vi "Error Query.vi"(0 "VISA Resource In":refnum<visa-resource-name>, 11 "error in (no error)":errorcluster) -> (4 "VISA Resource Out (dupl)":refnum<visa-resource-name>, 6 "Error Code":i32[](array[numeric]), 8 "Error Message":string, 15 "error out":errorcluster)   [LabVIEW 2025, in "My Current Source.lvlib"]
doc: "Queries the instrument for any errors in the instrument's error queue. It will continue to read errors until all errors have been read from the instrument. Any errors will be returned in the error out indicator."
uses:
  My Current Source.lvlib
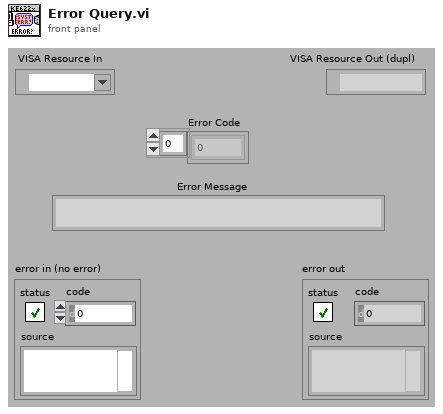
[diagram p1: front panel]
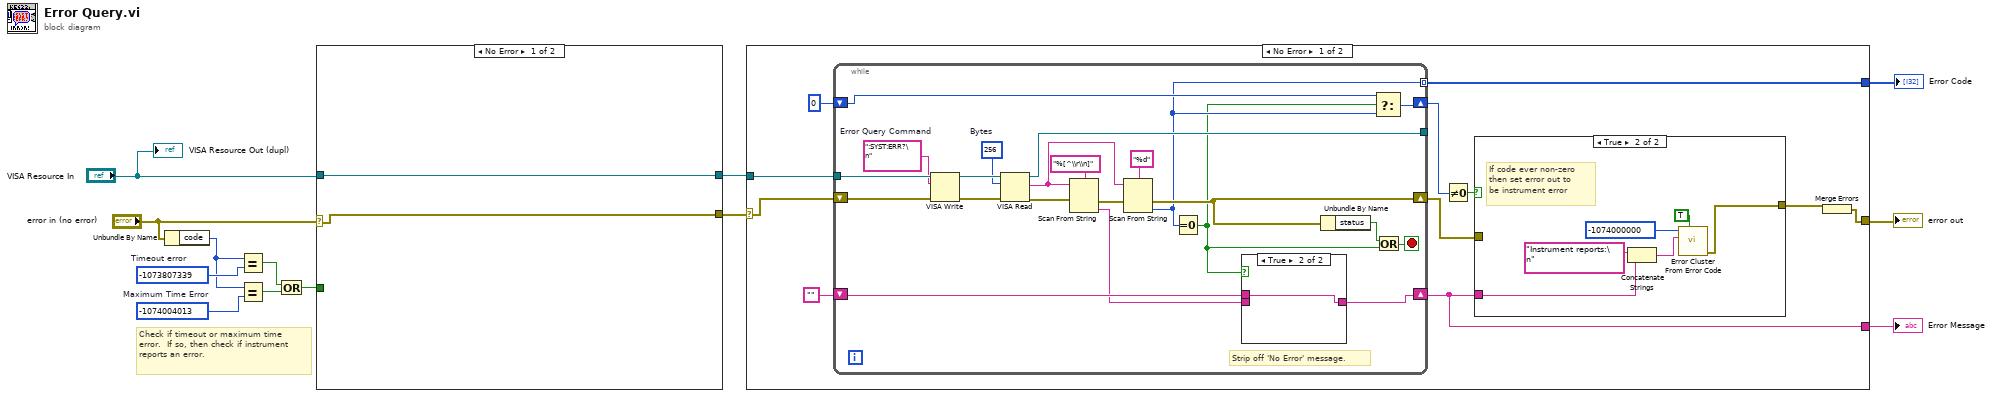
[diagram p0: block diagram]
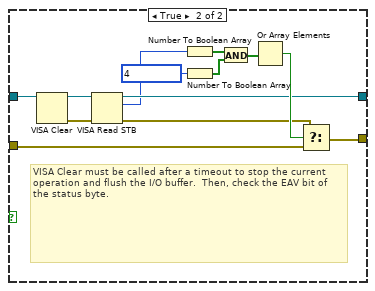
[diagram p3: hidden frame]
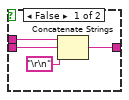
[diagram p5: hidden frame]
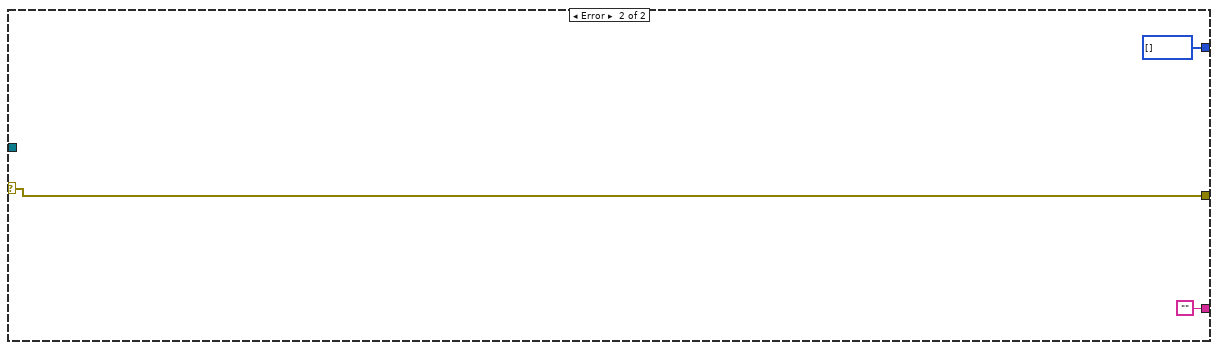
[diagram p6: hidden frame]
diagram:
  w6 = -1074004013  # Maximum Time Error
  w8 = -1073807339  # Timeout error
  # "Check if timeout or maximum time error.  If so, then check if instrument reports an error."
  n1 = Unbundle By Name("error in (no error)") -> ("code"=w7:i32)
  n2 = Equal?(x=w7, y=w8) -> (x = y?=w4:bool)
  n3 = Equal?(x=w7, y=w6) -> (x = y?=w5:bool)
  n4 = Or(x=w4, y=w5) -> (x .or. y?=w3:bool)
  n5 = case shown="No Error" "error in (no error)" {
    selector: "error in (no error)" -> [w14 w18]
    tunnel: "VISA Resource In" -> [w15 w20]
    tunnel: [w15 w19] -> w9
    tunnel: [w14 w17] -> w10
    tunnel: w3 -> [_ w16]
    frame No Error {
    }
    frame Error {
      n6 = case shown="False" w16 {
        tunnel: w20 -> [w22 w28]
        tunnel: [w22 w25] -> w19
        tunnel: w18 -> [w21 w31]
        tunnel: [w21 w30] -> w17
        frame False {
          # "Error code not a timeout, so best to pass on to user."
        }
        frame True {
          # "VISA Clear must be called after a timeout to stop the current operation and flush the I/O buffer.  Then, check the EAV bit of the status byte."
          n7 = VISA Clear(VISA resource name=w28) -> (VISA resource name out=w27:refnum<visa-resource-name>, error out=w26:errorcluster)  [unwired: 1 in]
          n8 = VISA Read STB(8:w26, 11:w27) -> (0:w24:errorcluster, 2:w23:u16, 3:w25:refnum<visa-resource-name>)
          n9 = Number To Boolean Array(number=w23) -> (Boolean array=w32:bool[])
          n10 = Number To Boolean Array(number=u8 4) -> (Boolean array=w34:bool[])
          n11 = And(x=w32, y=w34) -> (x .and. y?=w33:bool[])
          n12 = Or Array Elements(Boolean array=w33) -> (logical OR=w29:bool)
          n13 = Select(t=w24, s=w29, f=w31) -> (s? t:f=w30:errorcluster)
        }
      }
    }
  }
  n14 = case shown="No Error" w10 {
    selector: w10 -> [w36 w81]
    tunnel: w9 -> [w46 _]
    tunnel: [w44 w81] -> w13
    tunnel: [w39 ""] -> w12
    tunnel: [w38 i32[] []] -> w11
    frame No Error {
      n15 = while {
        tunnel: [w75] -> _
        tunnel: w46 -> [w74]
        shift-right: [w63] -> w39
        shift-left: "" -> [w65]
        shift-right: [w61] -> w40
        shift-left: 0 -> [w62]
        shift-right: [w59] -> w37
        shift-left: w36 -> [w60]
        tunnel: [w55] -> w38 mode=indexing
        stop <- w68 stop-if-true
        w72 = u32 256  # Bytes
        w70 = ":SYST:ERR?\n"  # Error Query Command
        # "Strip off 'No Error' message."
        n16 = VISA Write(VISA resource name=w74, write buffer=w70, error in (no error)=w60) -> (VISA resource name out=w73:refnum<visa-resource-name>, error out=w71:errorcluster)  [unwired: 1 out]
        n17 = VISA Read(VISA resource name=w73, byte count=w72, error in (no error)=w71) -> (VISA resource name out=w75:refnum<visa-resource-name>, read buffer=w66:string, error out=w58:errorcluster)  [unwired: 1 out]
        n18 = Scan From String(format string="%[^\\r\\n]", input string=w66, error in=w58) -> (error out=w57:errorcluster, output 1=w64:string)  [unwired: 1 in, 3 out]
        n19 = Scan From String(format string="%d", input string=w66, error in=w57) -> (error out=w59:errorcluster, output 1=w55:i32)  [unwired: 1 in, 3 out]
        n20 = Equal To 0?(x=w55) -> (x = 0?=w54:bool)
        n21 = case shown="True" w54 {
          tunnel: w65 -> [w79 w80]
          tunnel: w64 -> [w77 _]
          tunnel: [w76 w80] -> w63
          frame False {
            n22 = Concatenate Strings(w79, w77, "\r\n") -> (w76:string)
          }
          frame True {
          }
        }
        n23 = Unbundle By Name(w59) -> ("status"=w56:bool)
        n24 = Select(t=w62, s=w54, f=w55) -> (s? t:f=w61:i32)
        n25 = Or(x=w56, y=w54) -> (x .or. y?=w68:bool)
      }
      n26 = Not Equal To 0?(x=w40) -> (x != 0?=w42:bool)
      n27 = case shown="True" w42 {
        tunnel: w39 -> [_ w52]
        tunnel: [w47 w48] -> w41
        tunnel: w37 -> [w47 _]
        frame False {
        }
        frame True {
          # "If code ever non-zero\nthen set error out to\nbe instrument error"
          n28 = Concatenate Strings("Instrument reports:\n" ("Source"), w52) -> (w49:string)
          n29 = call <vilib>:"Error Cluster From Error Code.vi"("show call chain? (False)"=TRUE, "error message (\"\")"=w49, "error code (0)"=-1074000000 ("Code")) -> ("error out"=w48:errorcluster)  [unwired: 1 in, 5 out]
        }
      }
      n30 = Merge Errors(w41) -> (w44:errorcluster)
    }
    frame Error {
    }
  }
  "error out" <- w13
  "Error Message" <- w12
  "Error Code" <- w11
  "VISA Resource Out (dupl)" <- "VISA Resource In"
